vi "Escape Pattern String.vi"(10 "Input":string) -> (2 "Result":string)   [LabVIEW 2020, in "Stream.lvlib" / "URLPattern.lvclass"]
uses:
  URLPattern.lvclass
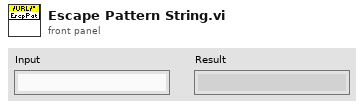
[diagram p1: front panel]
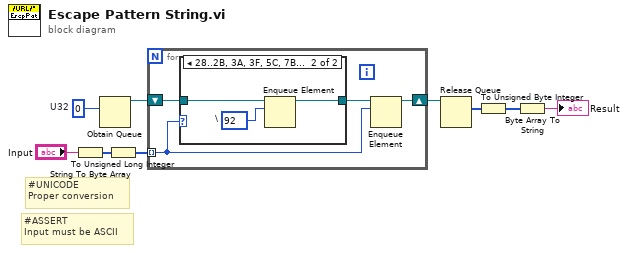
[diagram p0: block diagram]
diagram:
  w7 = u32 0  # U32
  # "#UNICODE\nProper conversion"
  # "#ASSERT\nInput must be ASCII"
  n1 = String To Byte Array(string="Input") -> (unsigned byte array=w8:u8[])
  n2 = Obtain Queue(element data type=w7) -> (queue out=w6:refnum<queue>)  [unwired: 4 in, 2 out]
  n3 = To Unsigned Long Integer(number=w8) -> (unsigned 32bit integer=w5:u32[])
  n4 = for {
    tunnel: w5 -> [w11] mode=indexing
    shift-right: [w10] -> w4
    shift-left: w6 -> [w13]
    n5 = case shown="28..2B, 3A, 3F, 5C, 7B, 7D" w11 {
      tunnel: w13 -> [w14 w17]
      tunnel: [w14 w16] -> w12
      frame Default {
      }
      frame 40..43, 58, 63, 92, 123, 125 {
        w15 = u32 92  # \
        n6 = Enqueue Element(queue=w17, element=w15) -> (queue out=w16:refnum<queue>)  [unwired: 2 in, 2 out]
      }
    }
    n7 = Enqueue Element(queue=w12, element=w11) -> (queue out=w10:refnum<queue>)  [unwired: 2 in, 2 out]
  }
  n8 = Release Queue(queue=w4) -> (remaining elements=w3:u32[])  [unwired: 2 in, 2 out]
  n9 = To Unsigned Byte Integer(number=w3) -> (unsigned 8bit integer=w2:u8[])
  n10 = Byte Array To String(unsigned byte array=w2) -> (string=→"Result":string)
